vi "EOL station.vi"(0 "configuration file path":path caption="配置文件的路径", 1 "EOL station msic inf":T1) -> ()   [LabVIEW 2014]
uses:
  Ctl.xio/EOL station msic ctl.ctl
  SubVIS.xio/DataSocket/DataSocket_Tags.ctl
  Ctl.xio/part type.ctl
  SubVIS.xio/Creat Write List VI's/DefCtrl/Station.ctl
  <vilib>/Utility/file.llb/Read From Spreadsheet File (string).vi
  SubVIS.xio/DataSocket/Read PLC Vars/Read Bool Var.vi
  SubVIS.xio/DataSocket/Read PLC Vars/Read U32 Var.vi
  SubVIS.xio/DataSocket/Write PLC Vars/Write Bool Var in.vi
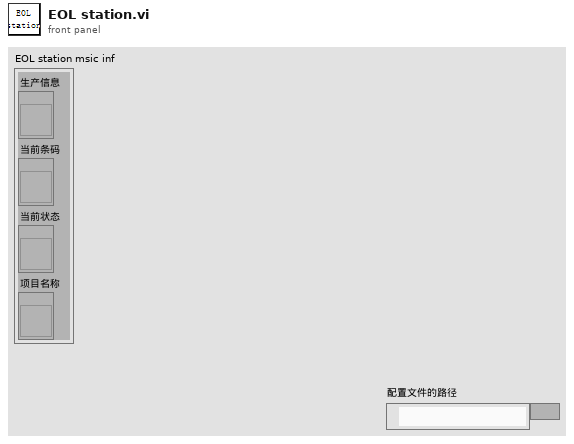
[diagram p1: front panel]
types:
  T1 = cluster{"生产信息":refnum<vi>, "当前条码":refnum<vi>, "当前状态":refnum<vi>, "项目名称":refnum<vi>}
  T2 = typedef "Station.ctl" = enum16{"粗切工位", "热处理工位", "精切工位", "PDF焊接工位", "打凹点预载力工位", "收卷工位", "EOL工位"}
  T3 = typedef "EOL station msic ctl.ctl" = cluster{"configuration file path":path, "DsOut":T4[], "Hopper car information":cluster{"Hopper car code":string, "Hopper car No":string, "plate No":string}, "pallet.produced number":i32, "SQL information":string, "Serial number":i32, "database path":path, "EOL station msic inf":cluster{"生产信息":refnum<vi>, "当前条码":refnum<vi>, "当前状态":refnum<vi>, "项目名称":refnum<vi>}, "part type":T5, "BarCode":string, "scanner resource name out":refnum<visa-resource-name>, "scanner coms":string, "Force value database":string[], "Force value buffer":dbl[], "SN":string, "print inf":string, "2Dcode inf":string, "Pass/Fail":bool}
  T4 = typedef "DataSocket_Tags.ctl" = cluster{"Ds ID":refnum<k13>, "Tag":string}
  T5 = typedef "part type.ctl" = cluster{"项目号":string, "物料代码":string, "零件号":string, "供应商编码":string, "产线编码":string, "客户代码":string, "颜色代码":string, "托盘上限":i32, "加热温度":string, "加热时长":string, "EOL Stations":string}
  T6 = cluster{"Hopper car code":string, "Hopper car No":string, "plate No":string}
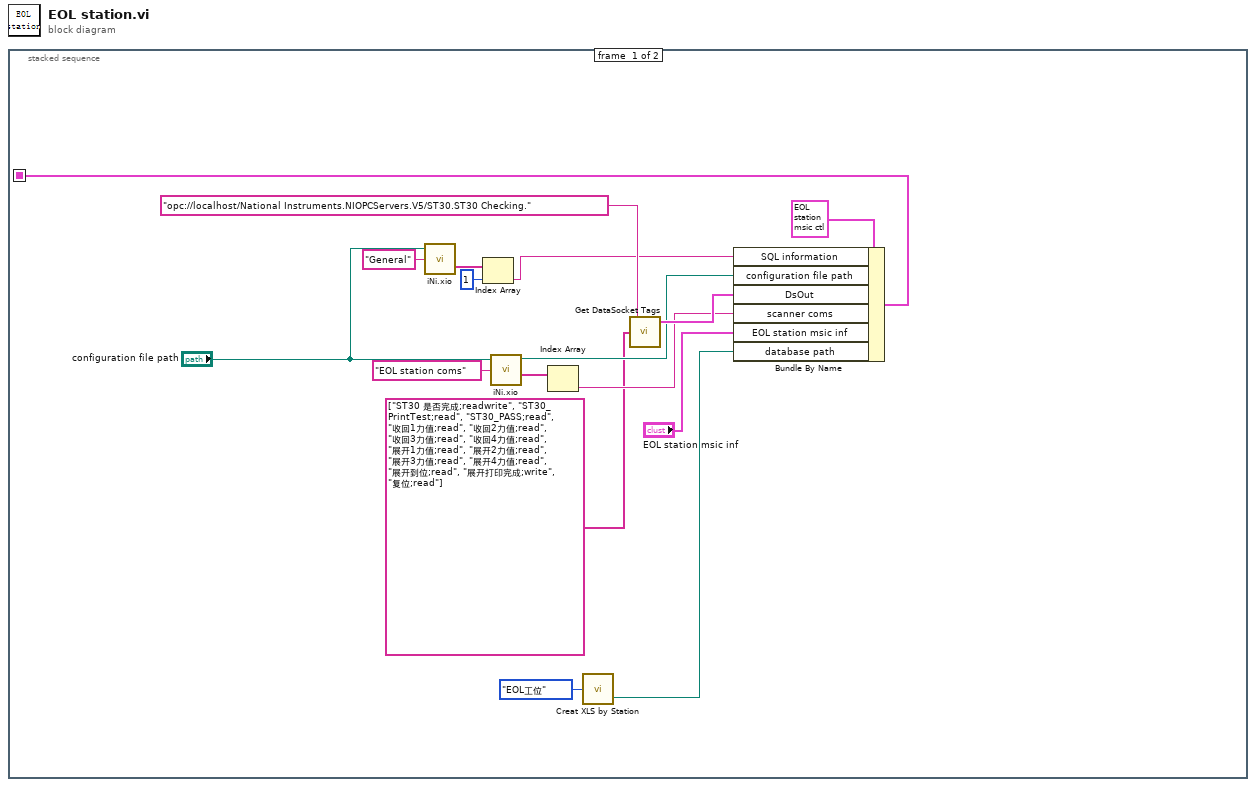
[diagram p0: block diagram]
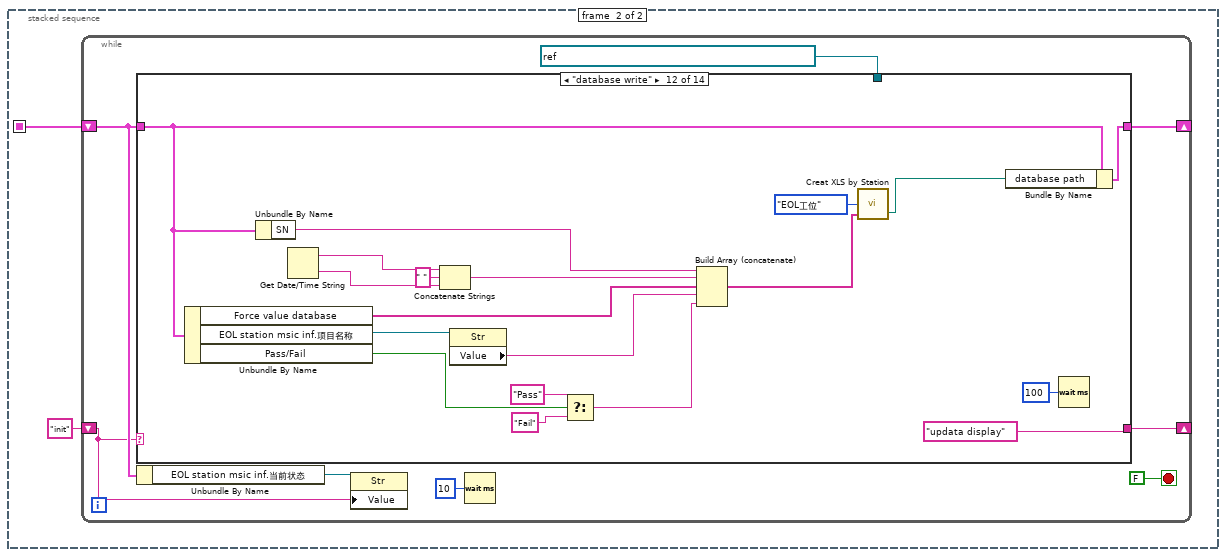
[diagram p2: hidden frame]
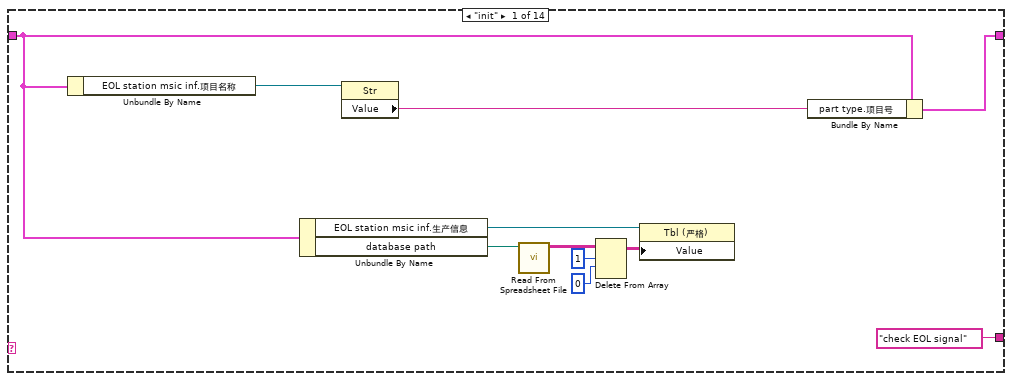
[diagram p3: hidden frame]
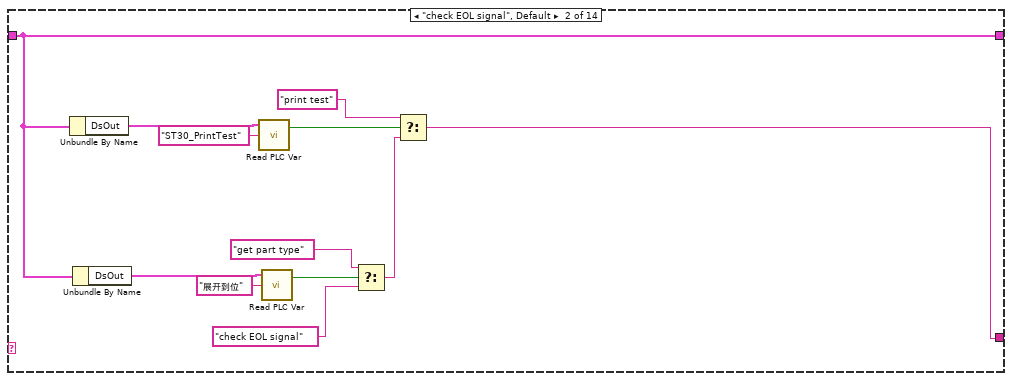
[diagram p4: hidden frame]
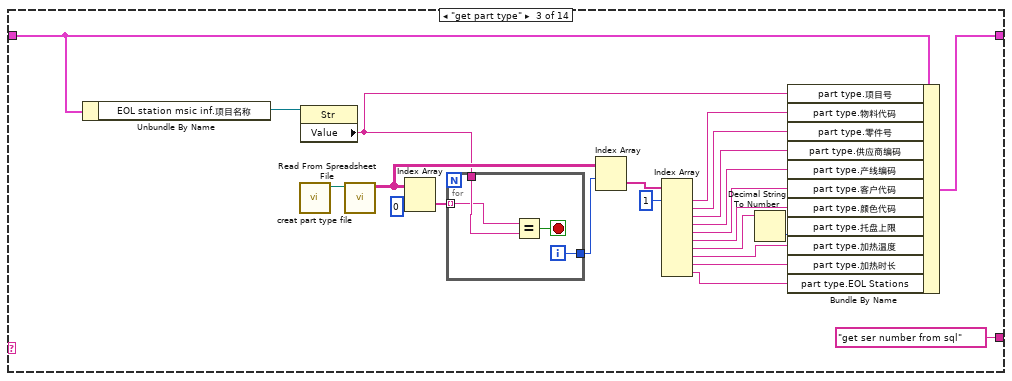
[diagram p5: hidden frame]
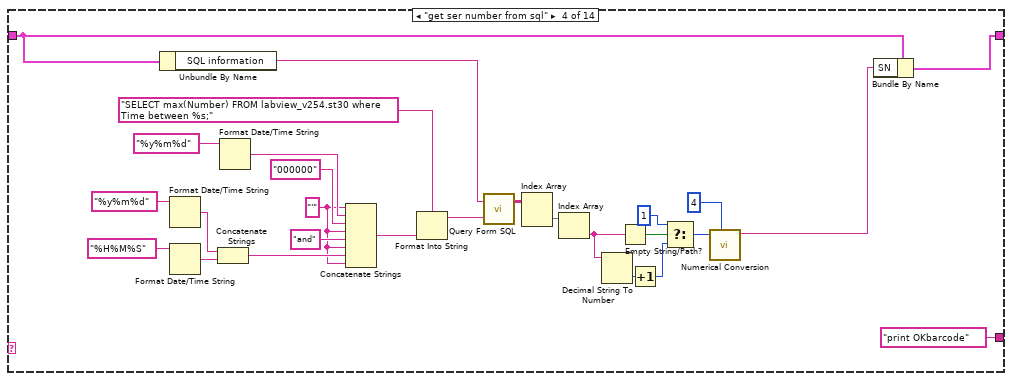
[diagram p6: hidden frame]
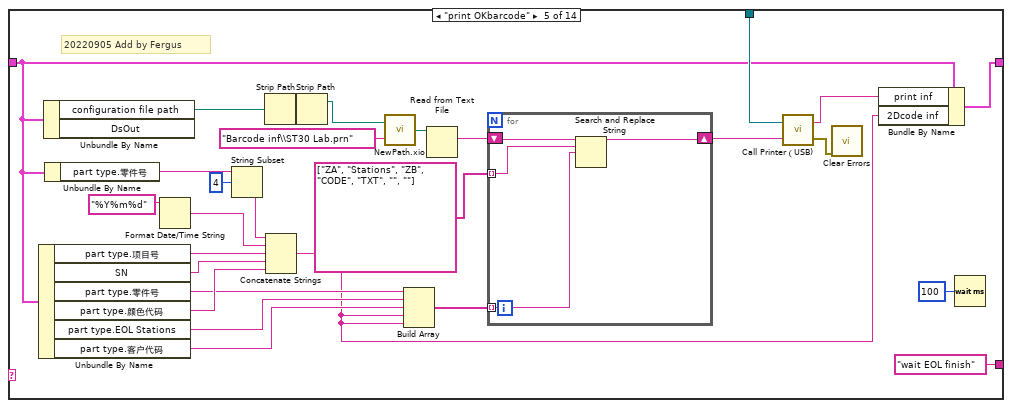
[diagram p7: hidden frame]
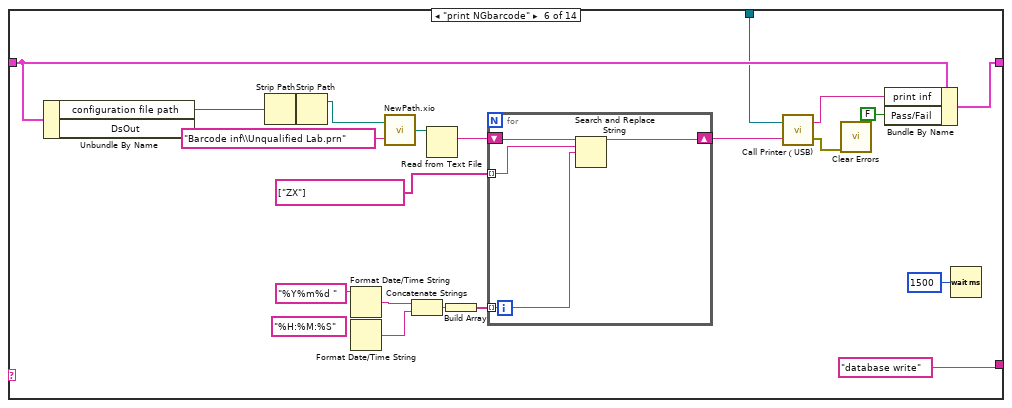
[diagram p8: hidden frame]
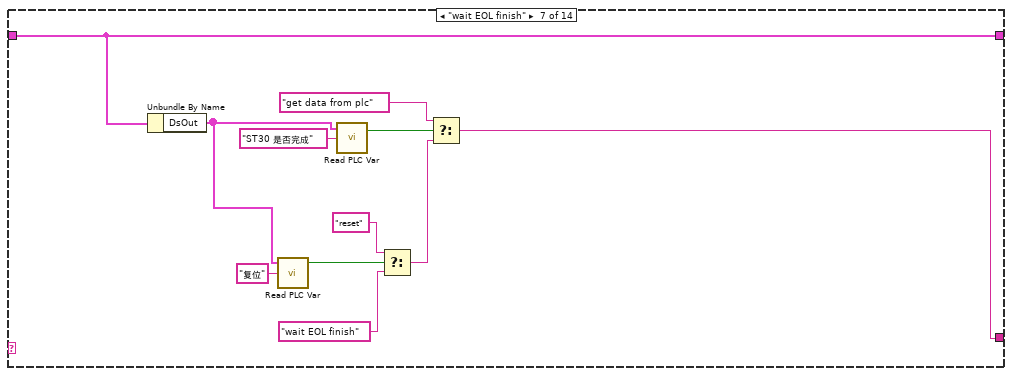
[diagram p9: hidden frame]
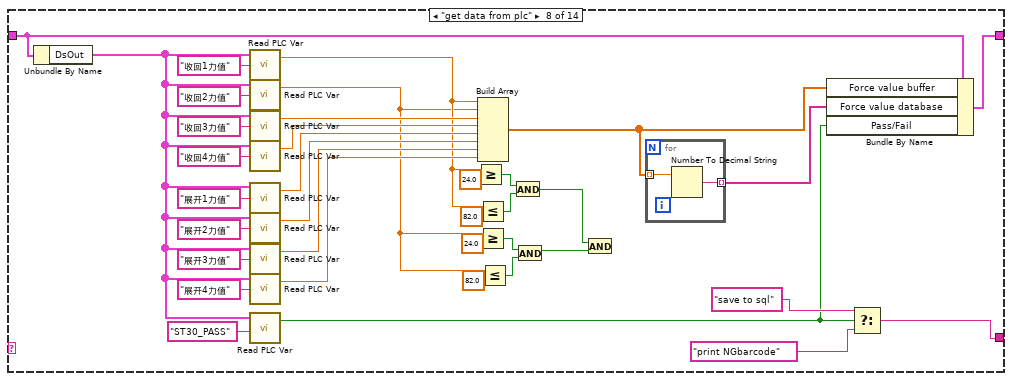
[diagram p10: hidden frame]
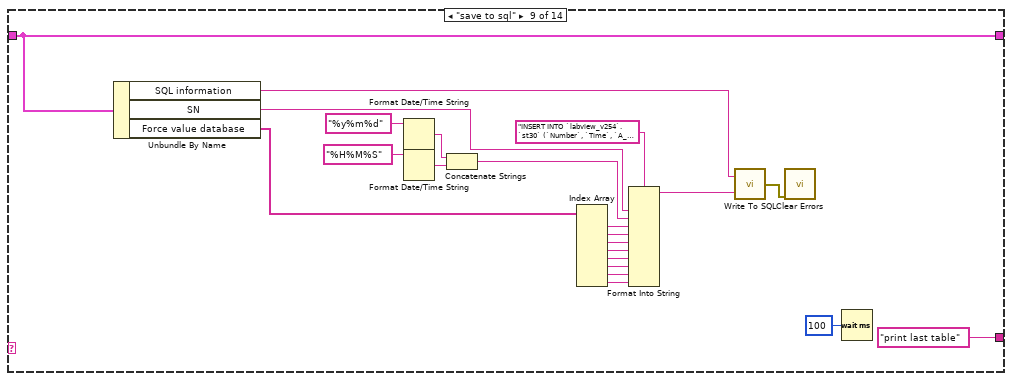
[diagram p11: hidden frame]
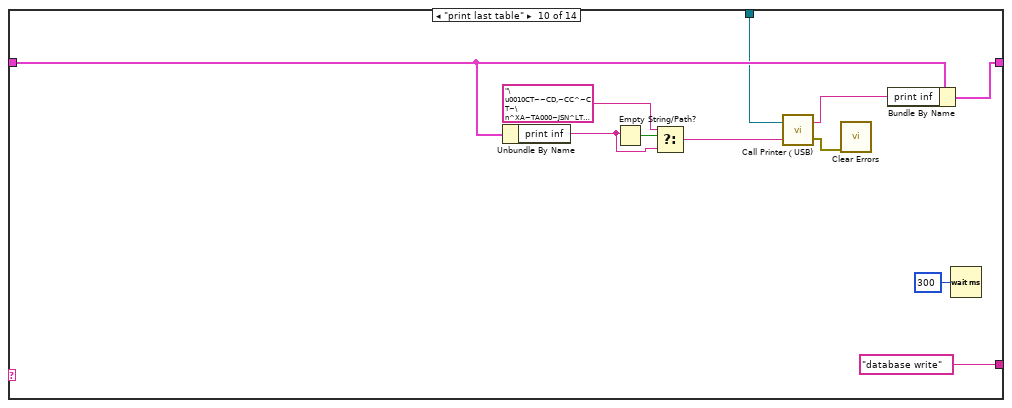
[diagram p12: hidden frame]
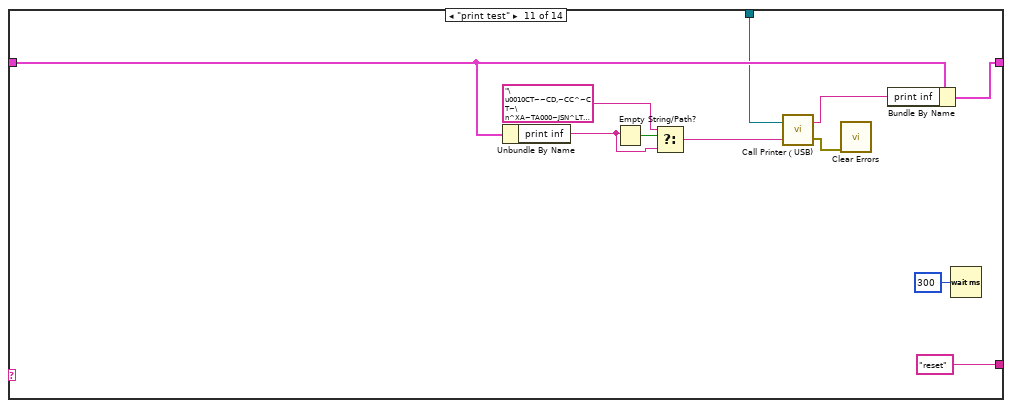
[diagram p13: hidden frame]
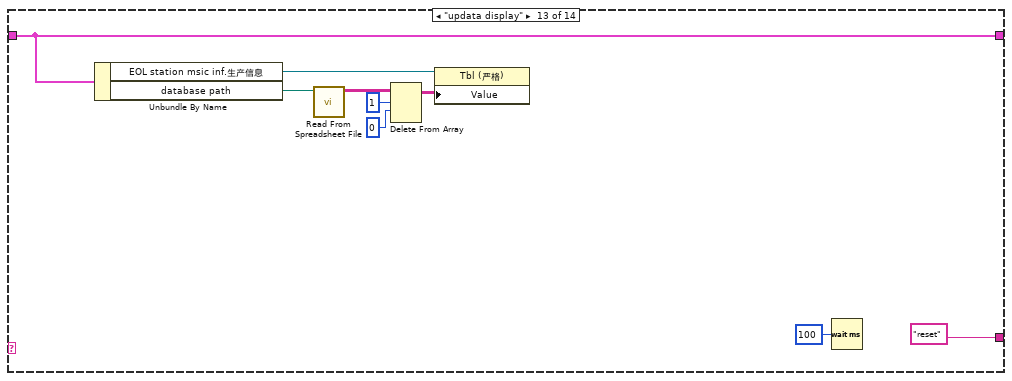
[diagram p14: hidden frame]
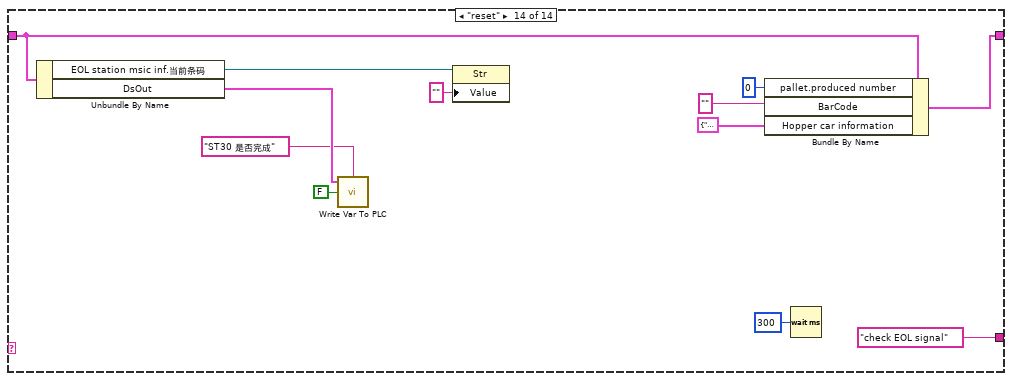
[diagram p15: hidden frame]
diagram:
  n1 = stacked-sequence {
    seq-local: [w10 _] -> [_ w18]
    frame #0 {
      n2 = call "iNi.xio.vi"("configuration file path"="configuration file path", "Sections"="General") -> ("Values"=w5:string[])  [unwired: 1 in, 4 out]
      n3 = Index Array(array=w5, index=1 ("索引")) -> (element=w3:string)
      n4 = call "iNi.xio.vi"("configuration file path"="configuration file path", "Sections"="EOL station coms") -> ("configuration file path"=w16:path, "Values"=w14:string[])  [unwired: 1 in, 3 out]
      n5 = Index Array(array=w14) -> (element=w13:string)  [unwired: 1 in]
      n6 = call "Creat XLS by Station.vi"("staiton"=Station."EOL工位") -> ("new file path (Not A Path if cancelled)"=w1:path)  [unwired: 5 in]
      n7 = call "Get DataSocket Tags.vi"("All Tags"=string[] ["ST30 是否完成;readwrite", "ST30_PrintTest;read", "ST30_PASS;read", "收回1力值;read", "收回2力值;read", "收回3力值;read", "收回4力值;read", "展开1力值;read", "展开2力值;read", "展开3力值;read", "展开4力值;read", "展开到位;read", "展开打印完成;write", "复位;read"], "URL"="opc://localhost/National Instruments.NIOPCServers.V5/ST30.ST30 Checking.") -> ("DsOut"=w17:T4[])  [unwired: 3 in]
      n8 = Bundle By Name(cluster=T3 {"configuration file path"=path "", "DsOut"=[], "Hopper car information"={"Hopper car code"="", "Hopper car No"="", "plate No"=""}, "pallet.produced number"=0, "SQL information"="", "Serial number"=0, "database path"=path "", "EOL station msic inf"={"生产信息"=refnum, "当前条码"=refnum, "当前状态"=refnum, "项目名称"=refnum}, "part type"={"项目号"="", "物料代码"="", "零件号"="", "供应商编码"="", "产线编码"="", "客户代码"="", "颜色代码"="", "托盘上限"=0, "加热温度"="", "加热时长"="", "EOL Stations"=""}, "BarCode"="", "scanner resource name out"="", "scanner coms"="", "Force value database"=[], "Force value buffer"=[], "SN"="", "print inf"="", "2Dcode inf"="", "Pass/Fail"=FALSE} ("PDF Welding msic ctl"), "SQL information"=w3, "configuration file path"=w16, "DsOut"=w17, "scanner coms"=w13, "EOL station msic inf"="EOL station msic inf", "database path"=w1) -> (w10:T3)
    }
    frame #1 {
      n9 = while {
        shift-right: [w27] -> _
        shift-left: w18 -> [w22]
        shift-right: [w26] -> _
        shift-left: "init" ("event") -> [w21]
        stop <- FALSE stop-if-true
        n10 = case shown="\"database write\"" w21 {
          tunnel: w22 -> [w28 w43 w72 w80 w108 w148 w169 w200 w213 w239 w250 w265 w280 w289]
          tunnel: [w38 w43 w51 w83 w113 w146 w169 w199 w213 w242 w253 w273 w280 w293] -> w27
          tunnel: ["check EOL signal" w39 "get ser number from sql" ("f") "print OKbarcode" ("f") "wait EOL finish" ("f") "database write" ("f") w168 w191 "print last table" ("f") "database write" ("f") "reset" ("f") "updata display" ("f") "reset" ("f") "check EOL signal" ("f")] -> w26
          tunnel: refnum<visa-resource-name> "USB0::0x0A5F::0x0081::29J194401307::RAW" ("VISA资源名称") -> [_ _ _ _ w109 w137 _ _ _ w233 w244 _ _ _]
          frame "init" {
            n11 = Unbundle By Name(w28) -> ("EOL station msic inf.项目名称"=w37:refnum<vi>)
            n12 = Unbundle By Name(w28) -> ("EOL station msic inf.生产信息"=w34:refnum<vi>, "database path"=w33:path)
            n13 = property class="Str"(reference=w37) -> ("Value"=w36:string)  [unwired: 1 in, 2 out]
            n14 = call-poly <vilib>:"Read From Spreadsheet File.vi"("file path (dialog if empty)"=w33) -> ("all rows"=w32:string[][])  [unwired: 6 in, 4 out]
            n15 = Delete From Array(array=w32, length=1 ("长度"), index (row)=0 ("索引 (行)")) -> (array with subset deleted=w29:string[][])  [unwired: 1 in, 1 out]
            n16 = property class="Tbl (严格)"(reference=w34, "Value"=w29) -> ()  [unwired: 1 in, 2 out]
            n17 = Bundle By Name(cluster=w28, "part type.项目号"=w36) -> (w38:T3)
          }
          frame "check EOL signal", Default {
            n18 = Unbundle By Name(w43) -> ("DsOut"=w44:T4[])
            n19 = Unbundle By Name(w43) -> ("DsOut"=w50:T4[])
            n20 = call-poly "Read PLC Var.vi"("Tag IN"="ST30_PrintTest", "Ds PLCTags IN"=w44) -> ("Bool Var out"=w42:bool)  [unwired: 1 in, 1 out]
            n21 = call-poly "Read PLC Var.vi"("Tag IN"="展开到位", "Ds PLCTags IN"=w50) -> ("Bool Var out"=w48:bool)  [unwired: 1 in, 1 out]
            n22 = Select(t="get part type" ("f"), s=w48, f="check EOL signal") -> (s? t:f=w41:string)
            n23 = Select(t="print test" ("f"), s=w42, f=w41) -> (s? t:f=w39:string)
          }
          frame "get part type" {
            n24 = Unbundle By Name(w72) -> ("EOL station msic inf.项目名称"=w73:refnum<vi>)
            n25 = call "creat part type file.vi"() -> ("new file path (Not A Path if cancelled)"=w66:path)  [unwired: 11 in]
            n26 = property class="Str"(reference=w73) -> ("Value"=w65:string)  [unwired: 1 in, 2 out]
            n27 = call-poly <vilib>:"Read From Spreadsheet File.vi"("file path (dialog if empty)"=w66) -> ("all rows"=w69:string[][])  [unwired: 6 in, 4 out]
            n28 = Index Array(array=w69, index (col)=0 ("禁用的索引 (列)")) -> (element=w70:string[])  [unwired: 1 in]
            n29 = for {
              tunnel: w70 -> [w74] mode=indexing
              tunnel: [w76] -> w68
              tunnel: w65 -> [w75]
              i -> [w76]
              stop <- w77 stop-if-true
              n30 = Equal?(x=w74, y=w75) -> (x = y?=w77:bool)
            }
            n31 = Index Array(array=w69, index (row)=w68) -> (element=w67:string[])  [unwired: 1 in]
            n32 = Index Array(array=w67, index #1=1 ("索引")) -> (element #1=w62:string, element #2=w61:string, element #3=w60:string, element #4=w59:string, element #5=w57:string, element #6=w58:string, element #7=w55:string, element #8=w54:string, element #9=w53:string, element #10=w52:string)  [unwired: 9 in]
            n33 = Decimal String To Number(string=w55) -> (number=w56:i32)  [unwired: 2 in, 1 out]
            n34 = Bundle By Name(cluster=w72, "part type.项目号"=w65, "part type.物料代码"=w62, "part type.零件号"=w61, "part type.供应商编码"=w60, "part type.产线编码"=w59, "part type.客户代码"=w57, "part type.颜色代码"=w58, "part type.托盘上限"=w56, "part type.加热温度"=w54, "part type.加热时长"=w53, "part type.EOL Stations"=w52) -> (w51:T3)
          }
          frame "get ser number from sql" {
            w94 = "'" ("字符串")
            n35 = Unbundle By Name(w80) -> ("SQL information"=w79:string)
            n36 = Format Date/Time String(time format string (%c)="%y%m%d" ("时间格式字符串(%c)")) -> (date/time string=w97:string)  [unwired: 2 in]
            n37 = Format Date/Time String(time format string (%c)="%H%M%S" ("时间格式字符串(%c)")) -> (date/time string=w98:string)  [unwired: 2 in]
            n38 = Concatenate Strings(w97, w98) -> (w95:string)
            n39 = Format Date/Time String(time format string (%c)="%y%m%d" ("时间格式字符串(%c)")) -> (date/time string=w101:string)  [unwired: 2 in]
            n40 = Concatenate Strings(w94, w101, "000000" ("字符串"), w94, "and" ("字符串"), w94, w95, w94) -> (w93:string)
            n41 = Format Into String(format string="SELECT max(Number) FROM labview_v254.st30 where Time between %s;" ("SQL query"), w93) -> (resulting string=w92:string)  [unwired: 2 in, 1 out]
            n42 = call "Query Form SQL.vi"("SQL query"=w92, "SQL ID"=w79) -> ("data"=w91:string[][])  [unwired: 1 out]
            n43 = Index Array(array=w91) -> (element=w90:string[])  [unwired: 2 in]
            n44 = Index Array(array=w90) -> (element=w86:string)  [unwired: 1 in]
            n45 = Decimal String To Number(string=w86) -> (number=w85:i32)  [unwired: 2 in, 1 out]
            n46 = Empty String/Path?(string/path=w86) -> (empty?=w89:bool)
            n47 = Increment(x=w85) -> (x+1=w84:i32)
            n48 = Select(t=1, s=w89, f=w84) -> (s? t:f=w87:i32)
            n49 = call "Numerical Conversion.vi"("width"=4, "num"=w87) -> ("字符串"=w82:string)  [unwired: 9 in]
            n50 = Bundle By Name(cluster=w80, "SN"=w82) -> (w83:T3)
          }
          frame "print OKbarcode" {
            # "20220905 Add by Fergus"
            n51 = Unbundle By Name(w108) -> ("part type.项目号"=w122:string, "SN"=w116:string, "part type.零件号"=w120:string, "part type.颜色代码"=w121:string, "part type.EOL Stations"=w119:string, "part type.客户代码"=w118:string)
            n52 = Unbundle By Name(w108) -> ("configuration file path"=w131:path)  [unwired: 1 out]
            n53 = Unbundle By Name(w108) -> ("part type.零件号"=w107:string)
            n54 = Format Date/Time String(time format string (%c)="%Y%m%d" ("时间格式字符串(%c)")) -> (date/time string=w123:string)  [unwired: 2 in]
            n55 = String Subset(string=w107, offset (0)=4 ("偏移量(0)")) -> (substring=w105:string)  [unwired: 1 in]
            n56 = Strip Path(path=w131) -> (stripped path=w130:path)  [unwired: 1 out]
            n57 = Concatenate Strings(w105, w123, w122, w116, w121) -> (w112:string)
            n58 = Strip Path(path=w130) -> (stripped path=w129:path)  [unwired: 1 out]
            n59 = call "NewPath.xio.vi"("Append path"="Barcode inf\\ST30 Lab.prn", "Basic path"=w129) -> ("New path"=w127:path)
            n60 = Build Array(w120, w119, w118, w112, w112) -> (w117:string[])
            n61 = Read from Text File(file (use dialog)=w127) -> (text=w126:string)  [unwired: 3 in, 3 out]
            n62 = for {
              shift-right: [w133] -> w115
              shift-left: w126 -> [w136]
              tunnel: string[] ["ZA", "Stations", "ZB", "CODE", "TXT", "", ""] -> [w135] mode=indexing
              tunnel: w117 -> [w134] mode=indexing
              n63 = Search and Replace String(input string=w136, search string=w135, replace string=w134) -> (result string=w133:string)  [unwired: 5 in, 3 out]
            }
            n64 = call "Call Printer（USB).vi"("写入缓冲区"=w115, "VISA资源名称"=w109) -> ("error out"=w111:errorcluster, "Last P"=w114:string)
            n65 = call <vilib>:"Clear Errors.vi"("error in (no error)"=w111) -> ()  [unwired: 5 in, 2 out]
            n66 = Bundle By Name(cluster=w108, "print inf"=w114, "2Dcode inf"=w112) -> (w113:T3)
            n67 = Wait (ms)(milliseconds to wait=u32 100 ("等待时间（毫秒）")) -> ()  [unwired: 1 out]
          }
          frame "print NGbarcode" {
            (unwired) "%H:%M:%S" ("时间格式字符串(%c)")
            n68 = Unbundle By Name(w148) -> ("configuration file path"=w157:path)  [unwired: 1 out]
            n69 = Strip Path(path=w157) -> (stripped path=w156:path)  [unwired: 1 out]
            n70 = Strip Path(path=w156) -> (stripped path=w155:path)  [unwired: 1 out]
            n71 = Format Date/Time String(time format string (%c)="%Y%m%d " ("时间格式字符串(%c)")) -> (date/time string=w144:string)  [unwired: 2 in]
            n72 = Format Date/Time String() -> (date/time string=w143:string)  [unwired: 3 in]
            n73 = call "NewPath.xio.vi"("Append path"="Barcode inf\\Unqualified Lab.prn", "Basic path"=w155) -> ("New path"=w153:path)
            n74 = Concatenate Strings(w144, w143) -> (w142:string)
            n75 = Read from Text File(file (use dialog)=w153) -> (text=w152:string)  [unwired: 3 in, 3 out]
            n76 = Build Array(w142) -> (w150:string[])
            n77 = for {
              shift-right: [w158] -> w149
              shift-left: w152 -> [w161]
              tunnel: string[] ["ZX"] -> [w160] mode=indexing
              tunnel: w150 -> [w159] mode=indexing
              n78 = Search and Replace String(input string=w161, search string=w160, replace string=w159) -> (result string=w158:string)  [unwired: 5 in, 3 out]
            }
            n79 = call "Call Printer（USB).vi"("写入缓冲区"=w149, "VISA资源名称"=w137) -> ("error out"=w141:errorcluster, "Last P"=w147:string)
            n80 = call <vilib>:"Clear Errors.vi"("error in (no error)"=w141) -> ()  [unwired: 5 in, 2 out]
            n81 = Bundle By Name(cluster=w148, "print inf"=w147, "Pass/Fail"=FALSE) -> (w146:T3)
            n82 = Wait (ms)(milliseconds to wait=u32 1500 ("等待时间（毫秒）")) -> ()  [unwired: 1 out]
          }
          frame "wait EOL finish" {
            n83 = Unbundle By Name(w169) -> ("DsOut"=w166:T4[])
            n84 = call-poly "Read PLC Var.vi"("Tag IN"="复位", "Ds PLCTags IN"=w166) -> ("Bool Var out"=w165:bool)  [unwired: 1 in, 1 out]
            n85 = call-poly "Read PLC Var.vi"("Tag IN"="ST30 是否完成", "Ds PLCTags IN"=w166) -> ("Bool Var out"=w171:bool)  [unwired: 1 in, 1 out]
            n86 = Select(t="reset" ("f"), s=w165, f="wait EOL finish") -> (s? t:f=w162:string)
            n87 = Select(t="get data from plc" ("f"), s=w171, f=w162) -> (s? t:f=w168:string)
          }
          frame "get data from plc" {
            n88 = Unbundle By Name(w200) -> ("DsOut"=w176:T4[])
            n89 = call-poly "Read PLC Var.vi"("Tag IN"="收回1力值", "Ds PLCTags IN"=w176) -> ("U32 Var out"=w187:dbl)  [unwired: 1 in, 1 out]
            n90 = call-poly "Read PLC Var.vi"("Tag IN"="收回2力值", "Ds PLCTags IN"=w176) -> ("U32 Var out"=w179:dbl)  [unwired: 1 in, 1 out]
            n91 = call-poly "Read PLC Var.vi"("Tag IN"="收回3力值", "Ds PLCTags IN"=w176) -> ("U32 Var out"=w198:dbl)  [unwired: 1 in, 1 out]
            n92 = call-poly "Read PLC Var.vi"("Tag IN"="收回4力值", "Ds PLCTags IN"=w176) -> ("U32 Var out"=w197:dbl)  [unwired: 1 in, 1 out]
            n93 = call-poly "Read PLC Var.vi"("Tag IN"="展开1力值", "Ds PLCTags IN"=w176) -> ("U32 Var out"=w193:dbl)  [unwired: 1 in, 1 out]
            n94 = call-poly "Read PLC Var.vi"("Tag IN"="展开2力值", "Ds PLCTags IN"=w176) -> ("U32 Var out"=w196:dbl)  [unwired: 1 in, 1 out]
            n95 = call-poly "Read PLC Var.vi"("Tag IN"="展开3力值", "Ds PLCTags IN"=w176) -> ("U32 Var out"=w195:dbl)  [unwired: 1 in, 1 out]
            n96 = call-poly "Read PLC Var.vi"("Tag IN"="展开4力值", "Ds PLCTags IN"=w176) -> ("U32 Var out"=w194:dbl)  [unwired: 1 in, 1 out]
            n97 = call-poly "Read PLC Var.vi"("Tag IN"="ST30_PASS", "Ds PLCTags IN"=w176) -> ("Bool Var out"=w173:bool)  [unwired: 1 in, 1 out]
            n98 = Greater Or Equal?(x=w187, y=24.0) -> (x >= y?=w184:bool)
            n99 = Build Array(w187, w179, w198, w197, w193, w196, w195, w194) -> (w190:dbl[])
            n100 = Less Or Equal?(x=w187, y=82.0) -> (x <= y?=w185:bool)
            n101 = Greater Or Equal?(x=w179, y=24.0) -> (x >= y?=w183:bool)
            n102 = Less Or Equal?(x=w179, y=82.0) -> (x <= y?=w182:bool)
            n103 = And(x=w184, y=w185) -> (x .and. y?=w177:bool)
            n104 = And(x=w183, y=w182) -> (x .and. y?=w178:bool)
            n105 = And(x=w177, y=w178) -> ()  [unwired: 1 out]
            n106 = for {
              tunnel: w190 -> [w210] mode=indexing
              tunnel: [w209] -> w189 mode=indexing
              n107 = Number To Decimal String(number=w210) -> (decimal integer string=w209:string)  [unwired: 1 in]
            }
            n108 = Bundle By Name(cluster=w200, "Force value buffer"=w190, "Force value database"=w189, "Pass/Fail"=w173) -> (w199:T3)
            n109 = Select(t="save to sql" ("f"), s=w173, f="print NGbarcode") -> (s? t:f=w191:string)
          }
          frame "save to sql" {
            n110 = Unbundle By Name(w213) -> ("SQL information"=w215:string, "SN"=w227:string, "Force value database"=w226:string[])
            n111 = Format Date/Time String(time format string (%c)="%y%m%d" ("时间格式字符串(%c)")) -> (date/time string=w230:string)  [unwired: 2 in]
            n112 = Format Date/Time String(time format string (%c)="%H%M%S" ("时间格式字符串(%c)")) -> (date/time string=w231:string)  [unwired: 2 in]
            n113 = Concatenate Strings(w230, w231) -> (w228:string)
            n114 = Index Array(array=w226) -> (element #1=w225:string, element #2=w224:string, element #3=w223:string, element #4=w222:string, element #5=w221:string, element #6=w220:string, element #7=w219:string, element #8=w218:string)  [unwired: 8 in]
            n115 = Format Into String(format string="INSERT INTO `labview_v254`.`st30` (`Number`, `Time`, `A_Data1`, `A_Data2`, `A_Data3`, `A_Data4`, `B_Data1`, `B_Data2`, `B_Data3`, `B_Data4`) VALUES ('%s', '%s', '%s', '%s', '%s', '%s', '%s', '%s', '%s', '%s');" ("初始字符串"), w227, w228, w225, w224, w223, w222, w221, w220, w219, w218) -> (resulting string=w216:string)  [unwired: 2 in, 1 out]
            n116 = call "Write To SQL.vi"("SQL query"=w216, "connection information"=w215) -> ("error out"=w214:errorcluster)
            n117 = call <vilib>:"Clear Errors.vi"("error in (no error)"=w214) -> ()  [unwired: 5 in, 2 out]
            n118 = Wait (ms)(milliseconds to wait=u32 100 ("等待时间（毫秒）")) -> ()  [unwired: 1 out]
          }
          frame "print last table" {
            n119 = Unbundle By Name(w239) -> ("print inf"=w236:string)
            n120 = Empty String/Path?(string/path=w236) -> (empty?=w238:bool)
            n121 = Select(t="\u0010CT~~CD,~CC^~CT~\n^XA~TA000~JSN^LT0^MNW^MTT^PON^PMN^LH0,0^JMA^PR5,5~SD15^JUS^LRN^CI0^XZ\n~DG000.GRF,00768,024,\n,::I07,I0780I0J8H0LA80H0E0I0380E,I0380I0IFE007FJF8001E0I0181C,02ABAA800EAAE002H2E228003F0I038380I0F0,07FIFC00C0060I01C0J0H3J0101FF80070,H0K8H0E00E0I01C0J0FBC0H0383AF800F0,H0701C0H0C0060I01C0J0E1C0017D7870H070,H0781E0H0E00E0I0380I03E0F003FHF870H0F0,H0301C0H0C0060I0780I0380780031DC70H070,H03C380H0IFE0I0F9C0H0F803E0078CEE0H0F0,J030P01FDE001E0H0FC07C07C0H070,0FJFE0N03B8F007BFHF3C0FE0380H0E0,07FIFE0N071870071J1H07F07E0H070,0E0K0HFEFFE00FB83C020L0HFBEFE00E0,070K0HFC7FE01C1C1E0M01F9F01E0060,0E0K0E0EE0E038380F003BHB803B9E00E0060,060K0C0C60607018070075H5C01907FF8,0E0K0E0EE0E0E0380200E001C03B838B8,0E0K0C0C6060H01C0I07001C01187018,0E0K0E0EE0E0H0380I0E001C00383038,1C0K0C0C6060H0180I07001C001070180070,1E0K0HFEFFE0H0380I0FAABC0038783800F0,1C0K0HFC7FE0H01C0I07FHFC00187D7800F0,380K0E0EE060H0380I0E003C00383AB8,30L040440J0180I07001C00107018,X080I0A0H0800282828,,::^XA\n^MMT\n^PW719\n^LL0096\n^LS0\n^FT166,88^A0N,20,21^FH\\^FDZX^FS\n^FT416,64^XG000.GRF,1,1^FS\n^FT78,88^A0N,20,21^FH\\^FDSerial nr:^FS\n^FT142,44^A0N,28,28^FH\\^FDNok^FS\n^PQ1,0,1,Y^XZ\n^XA^ID000.GRF^FS^XZ", s=w238, f=w236) -> (s? t:f=w235:string)
            n122 = call "Call Printer（USB).vi"("写入缓冲区"=w235, "VISA资源名称"=w233) -> ("error out"=w241:errorcluster, "Last P"=w243:string)
            n123 = call <vilib>:"Clear Errors.vi"("error in (no error)"=w241) -> ()  [unwired: 5 in, 2 out]
            n124 = Bundle By Name(cluster=w239, "print inf"=w243) -> (w242:T3)
            n125 = Wait (ms)(milliseconds to wait=u32 300 ("等待时间（毫秒）")) -> ()  [unwired: 1 out]
          }
          frame "print test" {
            n126 = Unbundle By Name(w250) -> ("print inf"=w247:string)
            n127 = Empty String/Path?(string/path=w247) -> (empty?=w249:bool)
            n128 = Select(t="\u0010CT~~CD,~CC^~CT~\n^XA~TA000~JSN^LT0^MNW^MTT^PON^PMN^LH0,0^JMA^PR5,5~SD15^JUS^LRN^CI0^XZ\n~DG000.GRF,00768,024,\n,::I07,I0780I0J8H0LA80H0E0I0380E,I0380I0IFE007FJF8001E0I0181C,02ABAA800EAAE002H2E228003F0I038380I0F0,07FIFC00C0060I01C0J0H3J0101FF80070,H0K8H0E00E0I01C0J0FBC0H0383AF800F0,H0701C0H0C0060I01C0J0E1C0017D7870H070,H0781E0H0E00E0I0380I03E0F003FHF870H0F0,H0301C0H0C0060I0780I0380780031DC70H070,H03C380H0IFE0I0F9C0H0F803E0078CEE0H0F0,J030P01FDE001E0H0FC07C07C0H070,0FJFE0N03B8F007BFHF3C0FE0380H0E0,07FIFE0N071870071J1H07F07E0H070,0E0K0HFEFFE00FB83C020L0HFBEFE00E0,070K0HFC7FE01C1C1E0M01F9F01E0060,0E0K0E0EE0E038380F003BHB803B9E00E0060,060K0C0C60607018070075H5C01907FF8,0E0K0E0EE0E0E0380200E001C03B838B8,0E0K0C0C6060H01C0I07001C01187018,0E0K0E0EE0E0H0380I0E001C00383038,1C0K0C0C6060H0180I07001C001070180070,1E0K0HFEFFE0H0380I0FAABC0038783800F0,1C0K0HFC7FE0H01C0I07FHFC00187D7800F0,380K0E0EE060H0380I0E003C00383AB8,30L040440J0180I07001C00107018,X080I0A0H0800282828,,::^XA\n^MMT\n^PW719\n^LL0096\n^LS0\n^FT166,88^A0N,20,21^FH\\^FDZX^FS\n^FT416,64^XG000.GRF,1,1^FS\n^FT78,88^A0N,20,21^FH\\^FDSerial nr:^FS\n^FT142,44^A0N,28,28^FH\\^FDNok^FS\n^PQ1,0,1,Y^XZ\n^XA^ID000.GRF^FS^XZ", s=w249, f=w247) -> (s? t:f=w246:string)
            n129 = call "Call Printer（USB).vi"("写入缓冲区"=w246, "VISA资源名称"=w244) -> ("error out"=w252:errorcluster, "Last P"=w254:string)
            n130 = call <vilib>:"Clear Errors.vi"("error in (no error)"=w252) -> ()  [unwired: 5 in, 2 out]
            n131 = Bundle By Name(cluster=w250, "print inf"=w254) -> (w253:T3)
            n132 = Wait (ms)(milliseconds to wait=u32 300 ("等待时间（毫秒）")) -> ()  [unwired: 1 out]
          }
          frame "database write" {
            n133 = Unbundle By Name(w265) -> ("Force value database"=w266:string[], "EOL station msic inf.项目名称"=w264:refnum<vi>, "Pass/Fail"=w261:bool)
            n134 = Unbundle By Name(w265) -> ("SN"=w272:string)
            n135 = Get Date/Time String() -> (date string=w269:string, time string=w268:string)  [unwired: 3 in]
            n136 = Concatenate Strings(w269, " " ("字符串"), w268) -> (w271:string)
            n137 = property class="Str"(reference=w264) -> ("Value"=w263:string)  [unwired: 1 in, 2 out]
            n138 = Select(t="Pass", s=w261, f="Fail") -> (s? t:f=w258:string)
            n139 = Build Array (concatenate)(w272, w271, w266, w263, w258) -> (w256:string[])
            n140 = call "Creat XLS by Station.vi"("staiton"=Station."EOL工位", "data in"=w256) -> ("new file path (Not A Path if cancelled)"=w255:path)  [unwired: 4 in]
            n141 = Bundle By Name(cluster=w265, "database path"=w255) -> (w273:T3)
            n142 = Wait (ms)(milliseconds to wait=u32 100 ("等待时间（毫秒）")) -> ()  [unwired: 1 out]
          }
          frame "updata display" {
            n143 = Unbundle By Name(w280) -> ("EOL station msic inf.生产信息"=w282:refnum<vi>, "database path"=w281:path)
            n144 = call-poly <vilib>:"Read From Spreadsheet File.vi"("file path (dialog if empty)"=w281) -> ("all rows"=w279:string[][])  [unwired: 6 in, 4 out]
            n145 = Delete From Array(array=w279, length=1 ("长度"), index (row)=0 ("索引 (行)")) -> (array with subset deleted=w276:string[][])  [unwired: 1 in, 1 out]
            n146 = property class="Tbl (严格)"(reference=w282, "Value"=w276) -> ()  [unwired: 1 in, 2 out]
            n147 = Wait (ms)(milliseconds to wait=u32 100 ("等待时间（毫秒）")) -> ()  [unwired: 1 out]
          }
          frame "reset" {
            n148 = Unbundle By Name(w289) -> ("EOL station msic inf.当前条码"=w288:refnum<vi>, "DsOut"=w285:T4[])
            n149 = call-poly "Write Var To PLC.vi"("Tag IN"="ST30 是否完成", "Bool Var in"=FALSE, "Ds PLCTags IN"=w285) -> ()  [unwired: 1 in, 2 out]
            n150 = property class="Str"(reference=w288, "Value"="" ("值")) -> ()  [unwired: 1 in, 2 out]
            n151 = Bundle By Name(cluster=w289, "pallet.produced number"=0, "BarCode"="", "Hopper car information"=T6 {"Hopper car code"="", "Hopper car No"="", "plate No"=""}) -> (w293:T3)
            n152 = Wait (ms)(milliseconds to wait=u32 300 ("等待时间（毫秒）")) -> ()  [unwired: 1 out]
          }
        }
        n153 = Unbundle By Name(w22) -> ("EOL station msic inf.当前状态"=w23:refnum<vi>)
        n154 = property class="Str"(reference=w23, "Value"=w21) -> ()  [unwired: 1 in, 2 out]
        n155 = Wait (ms)(milliseconds to wait=u32 10 ("等待时间（毫秒）")) -> ()  [unwired: 1 out]
      }
    }
  }
